vi "5TMonitor.vi"() -> ()   [LabVIEW 2019]
uses:
  Utility/Monitor Communication/Mischer/5T-Cluster.ctl
  Instrument_Setup.vi
  Global/Global Variables/Data_Display_global.vi
panel:
  out "5 T Cluster":T1 {"Rate (T/min)" format="%6_5f"; "Leads (T)" format="%6_5f"}
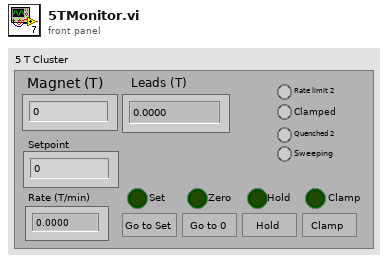
[diagram p1: front panel]
types:
  T1 = typedef "5T-Cluster.ctl" = cluster{"Go to set":bool, "Go to Zero":bool, "Clamp":bool, "Go to Hold":bool, "Clamped ":bool, "Quenched 2":bool, "Rate limit 2":bool, "Magnet (T)":dbl, "Leads (T)":dbl, "Rate (T/min)":dbl, "Sweeping":bool, "Setpoint":dbl, "Set":bool, "Zero":bool, "Hold":bool, "Clamp":bool}
  T2 = typedef "PSIO.ctl" = cluster{"Address":T3, "Version":enum16{"PS", "IPS"}}
  T3 = typedef "OxfordAddress.ctl" = cluster{"Com Port":i32, "ISOBUS Address":i32, "GPIB Address":i16, "Communication":enum16{"RS232", "ISOBUS", "GPIB", "Gateway"}}
  T4 = cluster{"Version\n":string, "Max Sweep":dbl[unit], "Max Field":dbl[unit], "IO Info":T2}
  T5 = cluster{"Value":i16, "At rest":bool, "Sweeping":bool, "Rate limiting":bool}
  T6 = cluster{"Value":i16, "Hold":bool, "To set point":bool, "To zero":bool, "Clamped":bool}
  T7 = cluster{"Value":i16, "Desired":u16, "Magnet":u16, "Commanded":u16, "Actual":u16}
  T8 = cluster{"Value":i16, "Quenched":bool, "Over heated":bool, "Warming up":bool}
  T9 = typedef "5T_Control.ctl" = cluster{"Rate (T/min)":dbl, "Setpoint":dbl, "Go to set":bool, "Go to Zero":bool, "Clamp":bool, "Go to Hold":bool, "Set Rate":bool}
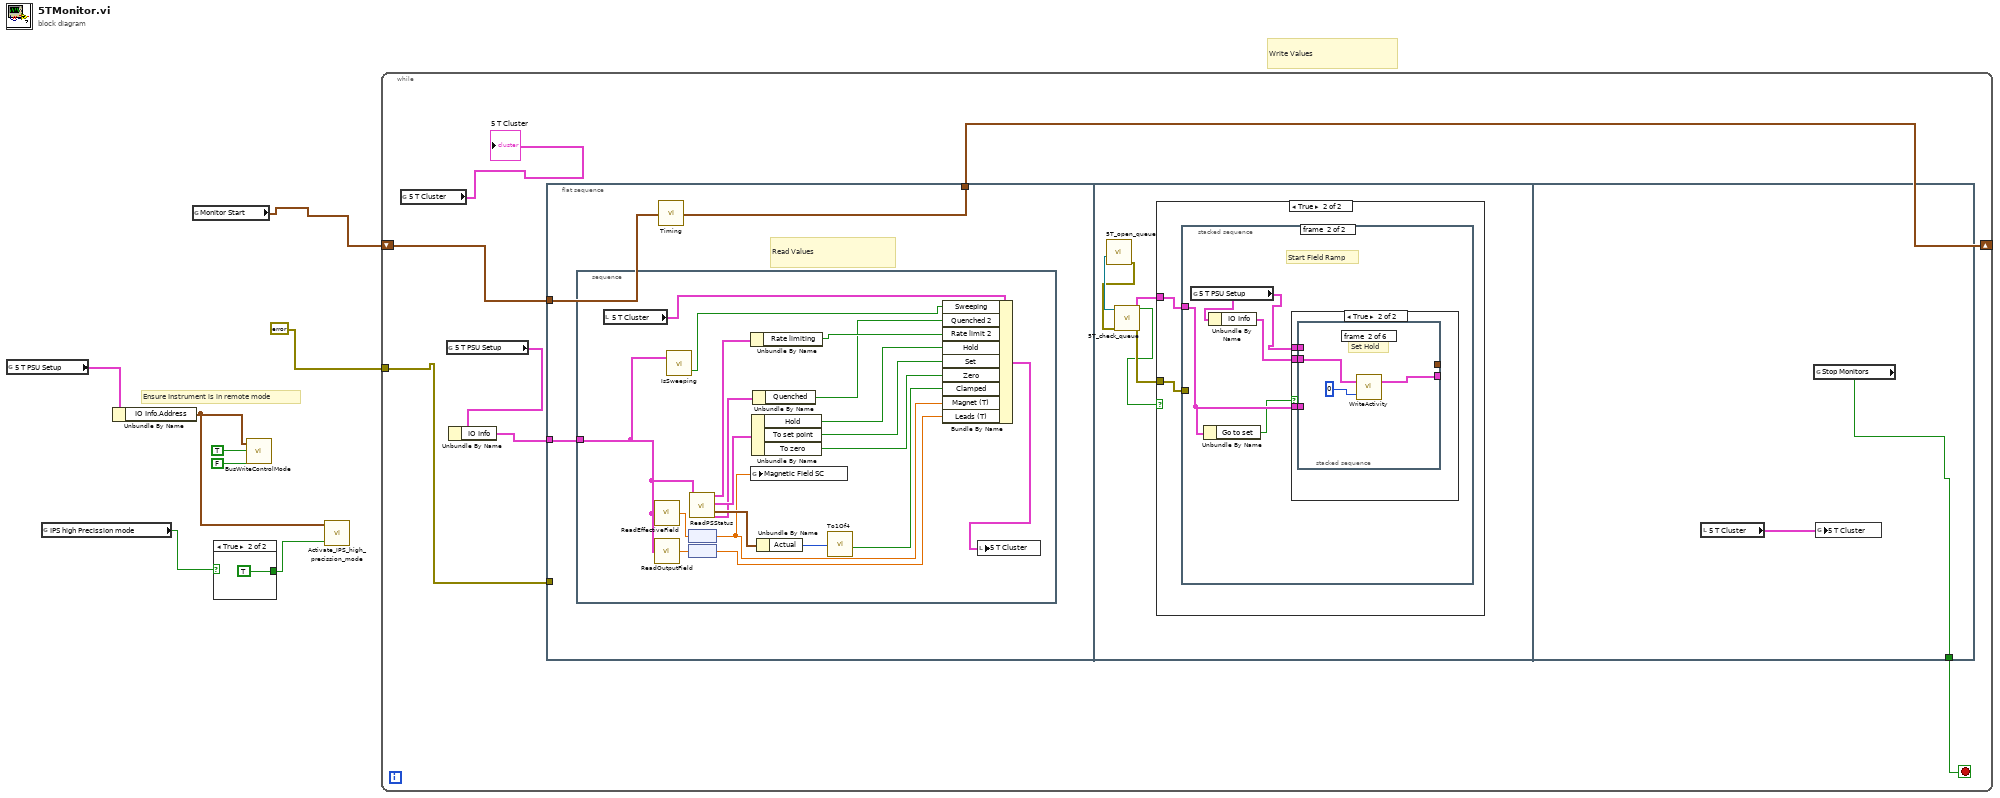
[diagram p0: block diagram]
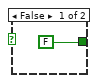
[diagram p2: hidden frame]
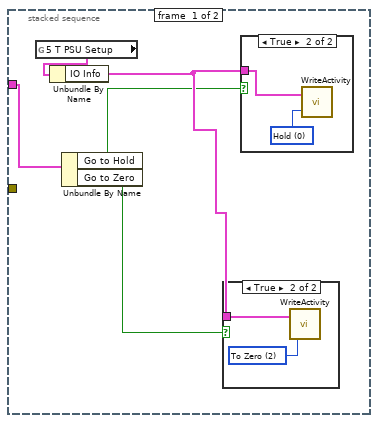
[diagram p4: hidden frame]
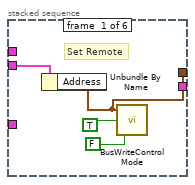
[diagram p8: hidden frame]
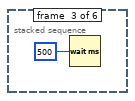
[diagram p9: hidden frame]
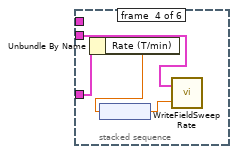
[diagram p10: hidden frame]
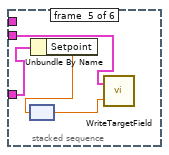
[diagram p11: hidden frame]
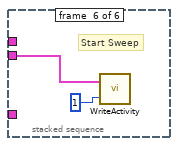
[diagram p12: hidden frame]
diagram:
  # "Ensure Instrument is in remote mode"
  # "Write Values"
  n1 = global read "Instrument_Setup.vi" "5 T PSU Setup"() -> (w7:T4)
  n2 = global read "Instrument_Setup.vi" "IPS high Precission mode"() -> (w2:bool)
  n3 = Unbundle By Name(w7) -> ("IO Info.Address"=w1:T3)
  n4 = global read "Data_Display_global.vi" "Monitor Start"() -> (w4:timestamp)
  n5 = case shown="True" w2 {
    tunnel: [FALSE TRUE] -> w3
    frame False {
    }
    frame True {
    }
  }
  n6 = call "BusWriteControlMode.vi"("Locked"=FALSE, "Remote"=TRUE, "Address"=w1) -> ()  [unwired: 1 out]
  n7 = call "Activate_IPS_high_precission_mode.vi"("High Precission"=w3, "Address"=w1) -> ()  [unwired: 1 in, 1 out]
  n8 = while {
    tunnel: errorcluster {"status"=FALSE, "code"=0, "source"=""} ("error constant") -> [w17]
    shift-right: [w15] -> _
    shift-left: w4 -> [w16]
    stop <- w14 stop-if-true
    n9 = global read "Data_Display_global.vi" "5 T Cluster"() -> (→"5 T Cluster":T1)
    n10 = global read "Instrument_Setup.vi" "5 T PSU Setup"() -> (w12:T4)
    n11 = Unbundle By Name(w12) -> ("IO Info"=w13:T2)
    n12 = flat-sequence {
      tunnel: w17 -> [_]
      tunnel: w16 -> [w19]
      tunnel: [w20] -> w15
      tunnel: w13 -> [w18]
      tunnel: [w82] -> w14
      frame #0 {
        # "Read Values"
        n13 = stacked-sequence {
          tunnel: w18 -> [w33]
          frame #0 {
            n14 = local read "5 T Cluster"() -> (w31:T1)
            n15 = call "ReadEffectiveField.vi"("IO Info"=w33) -> ("Effective field"=w34:dbl[unit])  [unwired: 2 out]
            n16 = call "ReadOutputField.vi"("IO Info"=w33) -> ("Field"=w35:dbl[unit])  [unwired: 2 out]
            n17 = call "IsSweeping.vi"("IO Info"=w33) -> ("Sweeping"=w28:bool)  [unwired: 1 in, 1 out]
            n18 = node(w34) -> (w22:dbl)
            n19 = node(w35) -> (w21:dbl)
            n20 = call "ReadPSStatus.vi"("IO Info"=w33) -> ("Mode (n)"=w38:T5, "Activity"=w39:T6, "Polarity"=w37:T7, "System Status (m)"=w36:T8)  [unwired: 10 in, 5 out]
            n21 = Unbundle By Name(w38) -> ("Rate limiting"=w29:bool)
            n22 = global write "Data_Display_global.vi" "Magnetic Field SC"(w22) -> ()
            n23 = Unbundle By Name(w39) -> ("Hold"=w26:bool, "To set point"=w25:bool, "To zero"=w24:bool)
            n24 = Unbundle By Name(w36) -> ("Quenched"=w27:bool)
            n25 = Unbundle By Name(w37) -> ("Actual"=w32:u16)
            n26 = call "To1Of4.vi"("Input"=w32) -> ("3"=w23:bool)  [unwired: 3 out]
            n27 = Bundle By Name(cluster=w31, "Sweeping"=w28, "Quenched 2"=w27, "Rate limit 2"=w29, "Hold"=w26, "Set"=w25, "Zero"=w24, "Clamped"=w23, "Magnet (T)"=w22, "Leads (T)"=w21) -> (w30:T1)
            n28 = local write "5 T Cluster"(w30) -> ()
          }
        }
        n29 = call "Timing.vi"("start time (s)"=w19) -> ("last reading (s)"=w20:timestamp)
      }
      frame #1 {
        n30 = call "5T_open_queue.vi"() -> ("error out"=w43:errorcluster, "queue out"=w44:refnum<queue>)  [unwired: 10 in]
        n31 = call "5T_check_queue.vi"("error in (no error)"=w43, "Queue"=w44) -> ("error out"=w42:errorcluster, "5T Control"=w41:T9, "New Entries?"=w40:bool)  [unwired: 6 in]
        n32 = case shown="True" w40 {
          tunnel: w42 -> [_ w46]
          tunnel: w41 -> [_ w45]
          frame False {
          }
          frame True {
            n33 = stacked-sequence {
              tunnel: w46 -> [_ _]
              tunnel: w45 -> [w49 w57]
              frame #0 {
                n34 = global read "Instrument_Setup.vi" "5 T PSU Setup"() -> (w51:T4)
                n35 = Unbundle By Name(w51) -> ("IO Info"=w50:T2)
                n36 = Unbundle By Name(w49) -> ("Go to Hold"=w48:bool, "Go to Zero"=w47:bool)
                n37 = case shown="True" w47 {
                  tunnel: w50 -> [_ w53]
                  frame False {
                  }
                  frame True {
                    w52 = u16 2 items=["Hold", "To Set Point", "To Zero", "Clamp"] ("Activity")
                    n38 = call "WriteActivity.vi"("Activity"=w52, "IO Info"=w53) -> ()  [unwired: 1 in, 1 out]
                  }
                }
                n39 = case shown="True" w48 {
                  tunnel: w50 -> [_ w55]
                  frame False {
                  }
                  frame True {
                    w54 = u16 0 items=["Hold", "To Set Point", "To Zero", "Clamp"] ("Activity")
                    n40 = call "WriteActivity.vi"("Activity"=w54, "IO Info"=w55) -> ()  [unwired: 1 in, 1 out]
                  }
                }
              }
              frame #1 {
                # "Start Field Ramp"
                n41 = global read "Instrument_Setup.vi" "5 T PSU Setup"() -> (w58:T4)
                n42 = Unbundle By Name(w57) -> ("Go to set"=w56:bool)
                n43 = Unbundle By Name(w58) -> ("IO Info"=w59:T2)
                n44 = case shown="True" w56 {
                  tunnel: w59 -> [_ w62]
                  tunnel: w58 -> [_ w61]
                  tunnel: w57 -> [_ w60]
                  frame False {
                  }
                  frame True {
                    n45 = stacked-sequence {
                      tunnel: [_ w69 _ _ _ _] -> _
                      tunnel: w62 -> [w64 w67 _ w73 w75 w79]
                      tunnel: [w63 _ _ _ _ _] -> _
                      tunnel: w61 -> [_ _ _ _ _ _]
                      tunnel: w60 -> [_ _ _ w74 w78 _]
                      frame #0 {
                        # "Set Remote"
                        n46 = Unbundle By Name(w64) -> ("Address"=w63:T3)
                        n47 = call "BusWriteControlMode.vi"("Locked"=FALSE, "Remote"=TRUE, "Address"=w63) -> ()  [unwired: 1 out]
                      }
                      frame #1 {
                        # "Set Hold"
                        n48 = call "WriteActivity.vi"("Activity"=0, "IO Info"=w67) -> ("IO Info"=w69:T2)  [unwired: 1 in]
                      }
                      frame #2 {
                        n49 = Wait (ms)(milliseconds to wait=u32 500) -> ()  [unwired: 1 out]
                      }
                      frame #3 {
                        n50 = Unbundle By Name(w74) -> ("Rate (T/min)"=w72:dbl)
                        n51 = node(w72) -> (w71:dbl[unit])
                        n52 = call "WriteFieldSweepRate.vi"("Sweep rate"=w71, "IO Info"=w73) -> ()  [unwired: 1 out]
                      }
                      frame #4 {
                        n53 = Unbundle By Name(w78) -> ("Setpoint"=w77:dbl)
                        n54 = node(w77) -> (w76:dbl[unit])
                        n55 = call "WriteTargetField.vi"("Target Field"=w76, "IO Info"=w75) -> ()  [unwired: 1 in, 1 out]
                      }
                      frame #5 {
                        # "Start Sweep"
                        n56 = call "WriteActivity.vi"("Activity"=1, "IO Info"=w79) -> ()  [unwired: 1 in, 1 out]
                      }
                    }
                  }
                }
              }
            }
          }
        }
      }
      frame #2 {
        n57 = local read "5 T Cluster"() -> (w81:T1)
        n58 = global read "Data_Display_global.vi" "Stop Monitors"() -> (w82:bool)
        n59 = global write "Data_Display_global.vi" "5 T Cluster"(w81) -> ()
      }
    }
  }
